vi "CellClicked--callback.vi"(4 "Args":refnum<user-event>, 5 "Event Data":cluster{"sender":refnum<k24>, "e":refnum<k24>}, 6 "Control Ref":refnum<k24>, 7 "Event Common Data":T1) -> ()   [LabVIEW 2025, in "FastTreeView.lvclass"]
uses:
  FastTreeView.lvclass
  FastTreeView.lvclass/FastTreeView.ctl
  C:/Git/FastTreeView/FastTreeView/LV/FastTreeView/dll/FastTreeView.dll
  dll/FastTreeView.dll
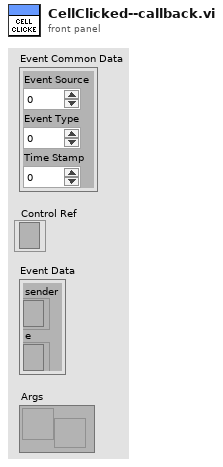
[diagram p1: front panel]
types:
  T1 = cluster{"Event Source":i32, "Event Type":u32, "Time Stamp":u32}
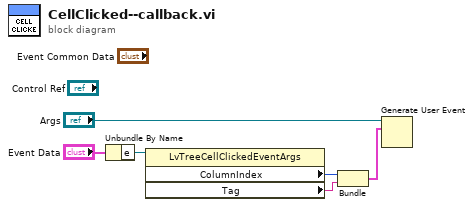
[diagram p0: block diagram]
diagram:
  n1 = Unbundle By Name("Event Data") -> ("e"=w4:refnum<k24>)
  n2 = property class="LvTreeCellClickedEventArgs"(reference=w4) -> ("ColumnIndex"=w3:i32, "Tag"=w2:string)  [unwired: 1 in, 2 out]
  n3 = Bundle("ColumnIndex"=w3, "Tag"=w2) -> (w1:cluster{"ColumnIndex":i32, "Tag":string})  [unwired: 1 in]
  n4 = Generate User Event(user event="Args", event data cluster=w1) -> ()  [unwired: 2 in, 2 out]
